vi "Init.vi"(5 "Autohide ListBox (F)":bool, 6 "Allow Undefined Values (F)":bool, 7 "ListBox Refnum (Popup)":refnum<vi>, 8 "error in (no error)":errorcluster, 9 "Height (200)":i16=200, 10 "Initial Options (Empty)":string[](array[string]), 11 "Str Refnum":refnum<vi>) -> (0 "error out":errorcluster, 3 "AutoComplete out":refnum<class "AutoComplete.lvclass">)   [LabVIEW 2020, in "AutoComplete.lvlib" / "AutoComplete.lvclass"]
doc: "Creates an AutoComplete handler wrapped in a class. This provides clearer APIs for how to interact with a running autocomplete handler.\n\n<b>Str Refnum</b> - The control that drives the search functionality and has the result placed in.\n<b>Initial Options</b> - The starting list of possible selections. This can bae updated later by generating a New Options event.\n<b>Height</b> - Sets the pixel height of the popup list when typing into the specified string.\n<b>ListBox Refnum</b> - Alternatively a separate ListBox can be specified that is integrated into the UI.\n<b>Autohide ListBox</b> - When specifying an external ListBox, this causes the listbox to be hidden whenever a selection is made.\n<b>Allow Undefined Values</b> - Allows users to enter arbitrary values in addition to what is available in the options list."
uses:
  AutoComplete.lvclass
  AutoComplete.lvclass/AutoComplete.ctl
  AutoComplete.lvlib
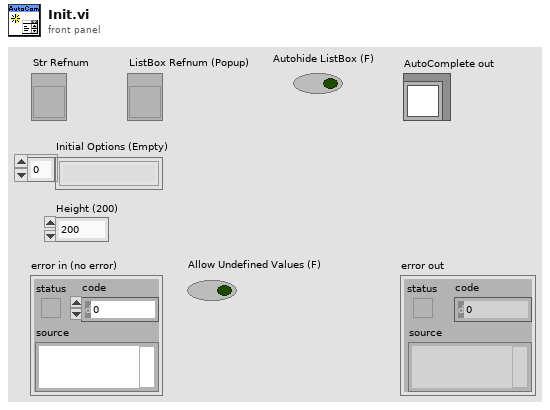
[diagram p1: front panel]
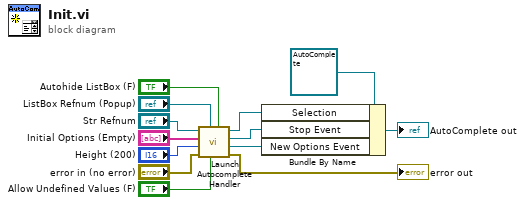
[diagram p0: block diagram]
diagram:
  n1 = call "Launch Autocomplete Handler.vi"("Autohide ListBox (F)"="Autohide ListBox (F)", "Allow Undefined Values (F)"="Allow Undefined Values (F)", "ListBox Refnum (Popup)"="ListBox Refnum (Popup)", "error in (no error)"="error in (no error)", "Height (200)"="Height (200)", "Initial Options (Empty)"="Initial Options (Empty)", "Str Refnum"="Str Refnum") -> ("error out"=→"error out":errorcluster, "New Options Event"=w3:refnum<user-event>, "Stop Event"=w4:refnum<user-event>, "Selection"=w5:refnum<user-event>)  [unwired: 1 in]
  n2 = Bundle By Name(cluster=refnum<class "AutoComplete.lvclass"> refnum ("AutoComplete in"), "Selection"=w5, "Stop Event"=w4, "New Options Event"=w3) -> (→"AutoComplete out":refnum<class "AutoComplete.lvclass">)
